vi "Pressure_4_R2.vi"() -> ()   [LabVIEW 2020]
uses:
  Support/Controls/Cmd_Mouse Popup.ctl
  Support/Controls/Clst_Initialize Input.ctl
  Support/Controls/Clst_Result inspec.ctl
  Support/Controls/Cmd_Var Data IO.ctl
  Variables/Global_Cal Info.vi
panel:
  in  "설정온도(℃)":string
  in  "측정시간(분)":string
  in  "STD Measured":string[][](table) caption="데이터로거 지시값 (bar)"
  out "Resolution":string[][](table) caption="Spec"
  in  "지시형태":string(combo)="Check"
  in  "Spec 변경":bool
  in  "Random":bool
  out "Spec":string[][](table)
  out "제목":string
  out "에러 출력":errorcluster
  out "Condition":string[][](table)
  in  "최소눈금":string(combo)
  out "단위":string
  in  "Measured":string[][](table) caption="교정대상기기 지시값"
  out "Load?":bool
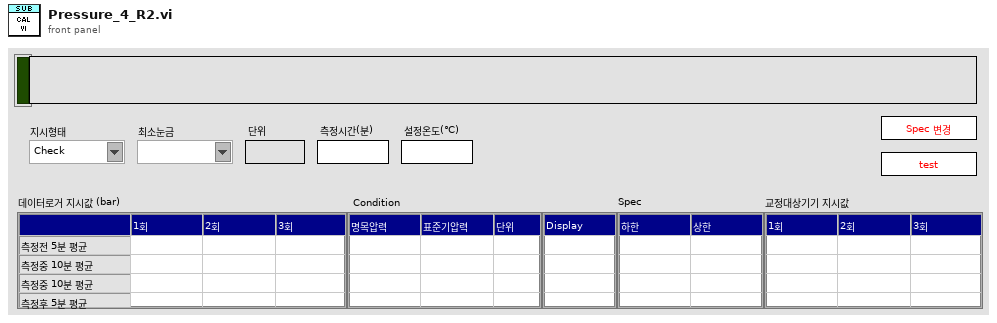
[diagram p1: front panel]
types:
  T1 = typedef "Cmd_Mouse Popup.ctl" = enum16{"활성화", "메뉴선택"}
  T2 = cluster{"Shift":bool, "Ctrl":bool, "Alt":bool, "Cmd":bool, "Opt":bool}
  T3 = typedef "Clst_Initialize Input.ctl" = cluster{"Initialize 1":cluster{"Condition":refnum<vi>[], "Spec":refnum<vi>[], "Measured":refnum<vi>[], "Resolution":refnum<vi>[], "Func_ext":string, "제목":refnum<vi>, "Measured_ADJ":refnum<vi>[]}, "Initialize 2":cluster{"문자열":refnum<vi>[], "콤보박스":refnum<vi>[], "링":refnum<vi>[], "열거형":refnum<vi>[], "테이블":refnum<vi>[], "여러열":refnum<vi>[], "디지털(DBL)":refnum<vi>[], "3D string":refnum<vi>[], "ctrl":refnum<vi>[], "boolean":refnum<vi>[]}}
  T4 = typedef "Clst_Result inspec.ctl" = cluster{"분해능":string, "문자열 1":string, "문자열 2":string, "숫자형 1":i32, "숫자형 2":i32, "숫자형 3":dbl, "문자배열 1D":string[], "문자배열 2D":string[][], "문자배열 3D":string[][][], "문자배열 4D":string[][][][], "불리언 1D":bool[]}
  T5 = typedef "Cmd_Var Data IO.ctl" = enum16{"Condition", "Condition Default", "Condition_Temp", "Resolution", "Resolution Default", "Resolution Old", "Spec", "Spec Default", "Spec Old", "Spec Temp", "Result", "Result2", "Result3", "Result_Temp", "Result_ADJ", "Result_ADJ2", "STD1", "STD2", "STD3", "STD4", "STD5", "STD Temp", "CMC", "CMC Default"}
  T6 = enum8{"Enabled", "Disabled", "Disabled and Grayed Out"}
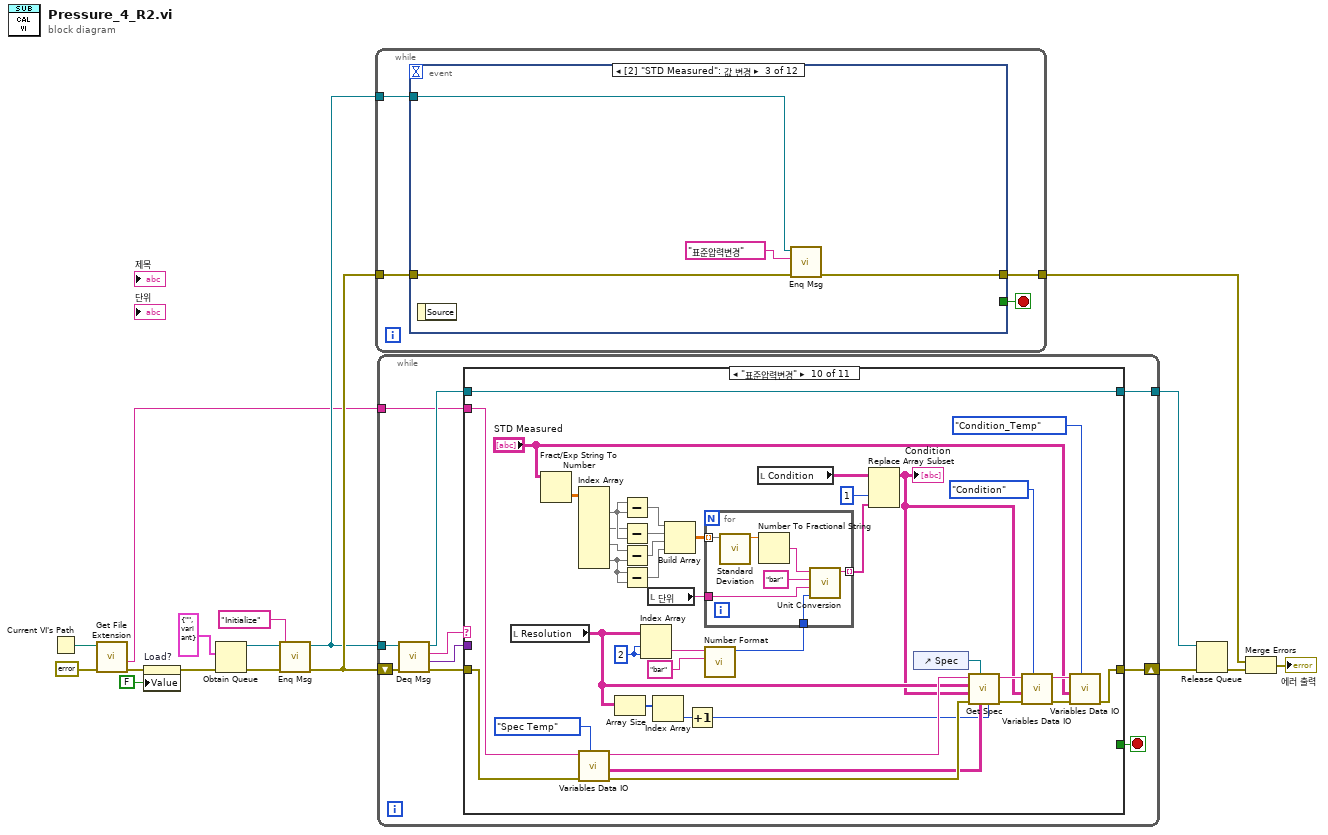
[diagram p0: block diagram]
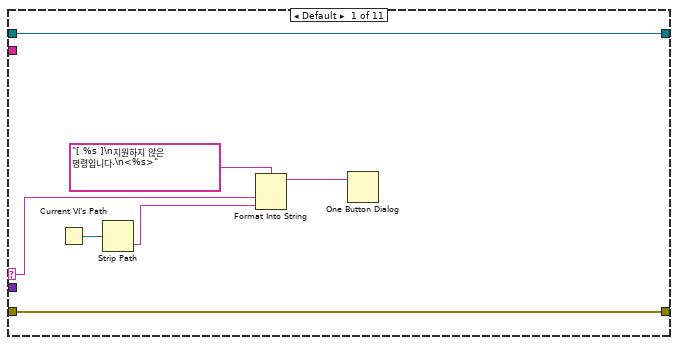
[diagram p2: hidden frame]
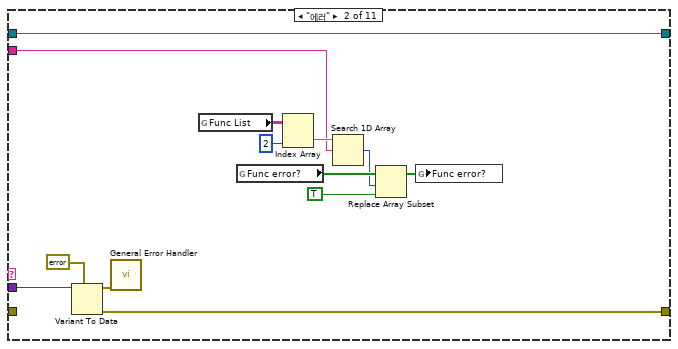
[diagram p3: hidden frame]
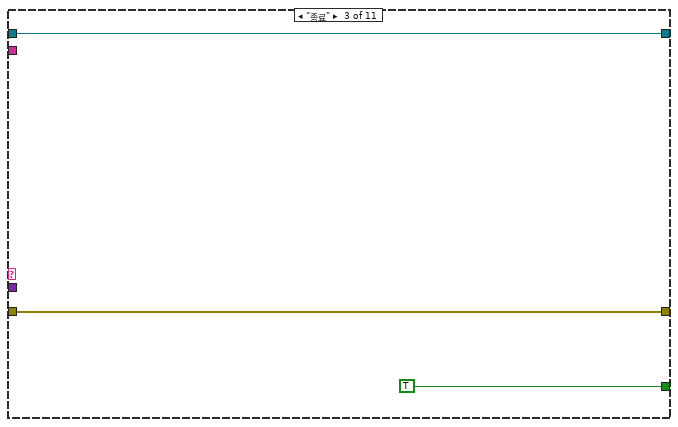
[diagram p4: hidden frame]
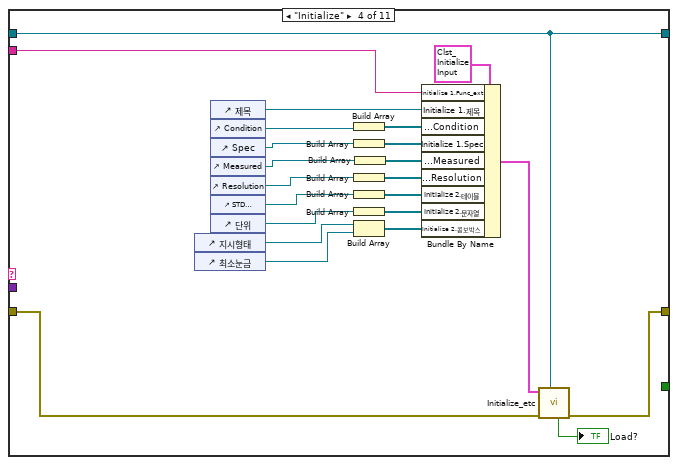
[diagram p5: hidden frame]
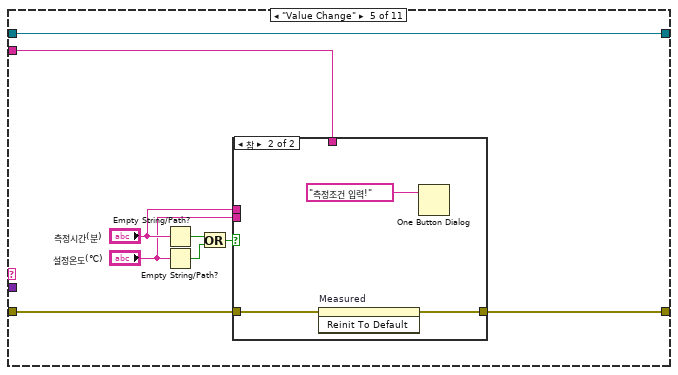
[diagram p6: hidden frame]
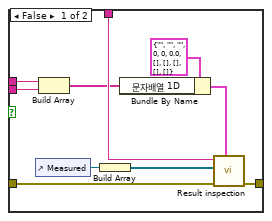
[diagram p7: hidden frame]
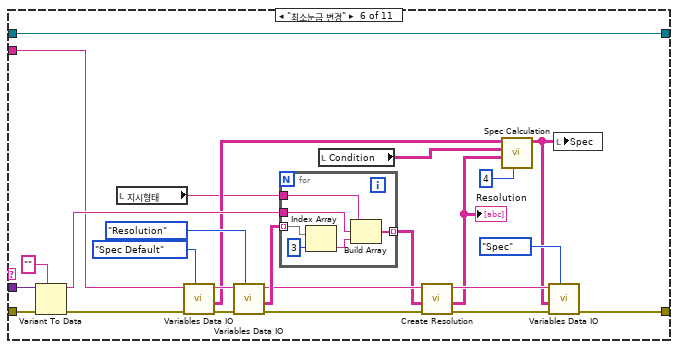
[diagram p8: hidden frame]
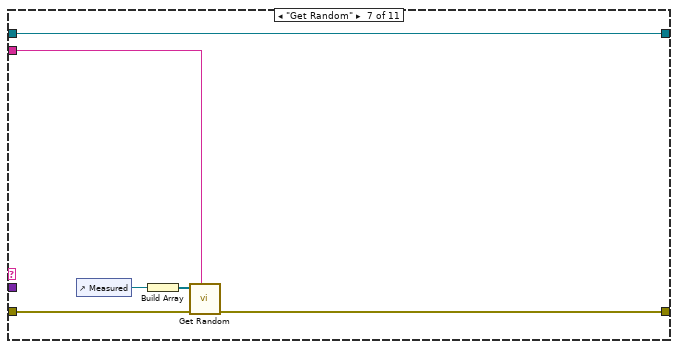
[diagram p9: hidden frame]
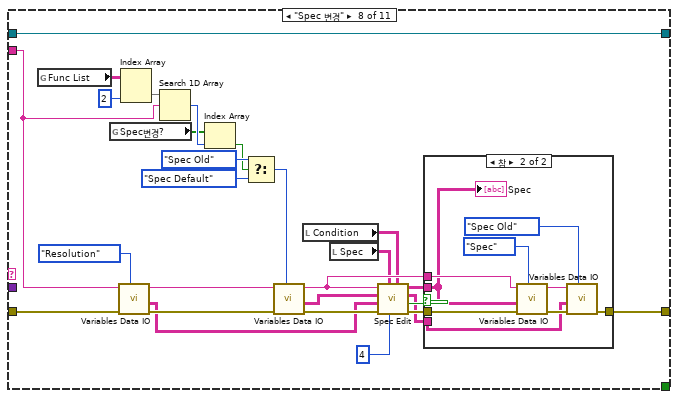
[diagram p10: hidden frame]
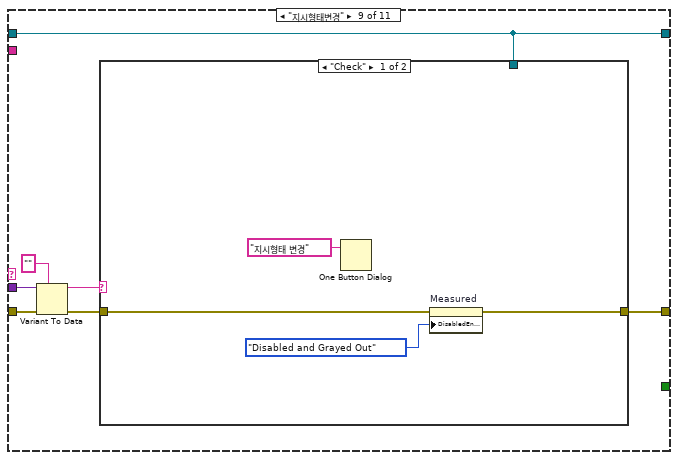
[diagram p12: hidden frame]
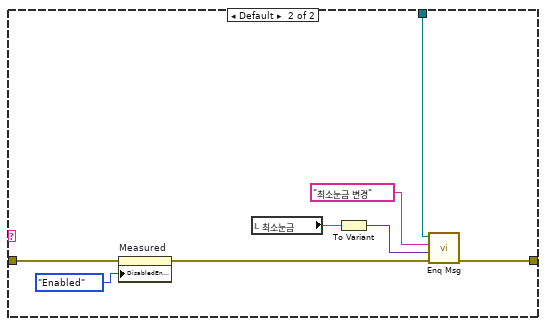
[diagram p13: hidden frame]
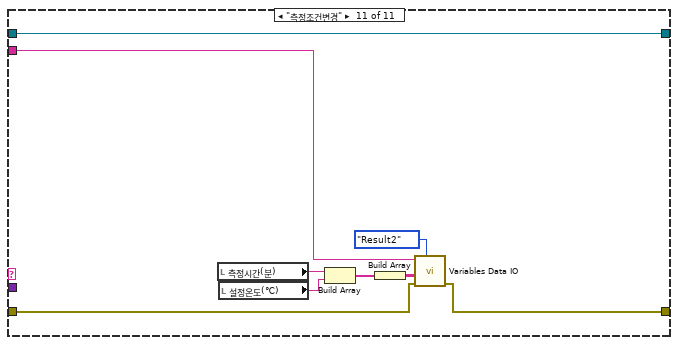
[diagram p14: hidden frame]
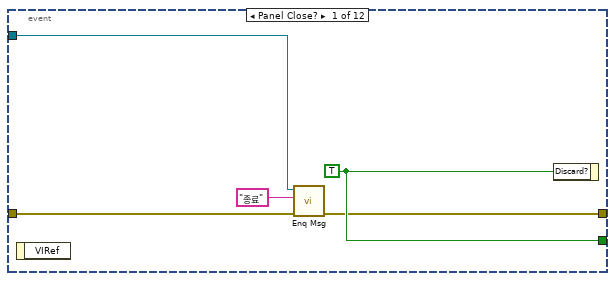
[diagram p15: hidden frame]
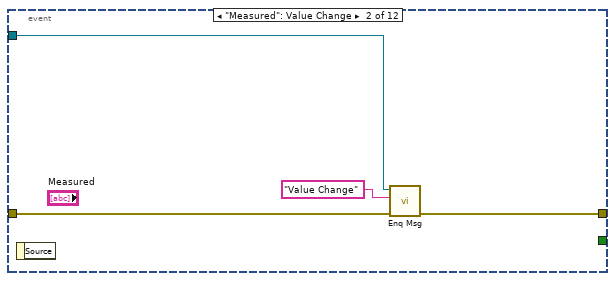
[diagram p16: hidden frame]
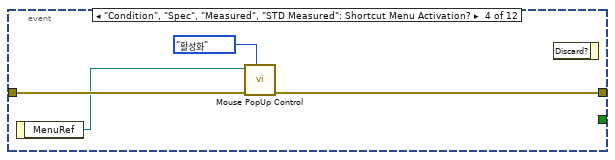
[diagram p17: hidden frame]
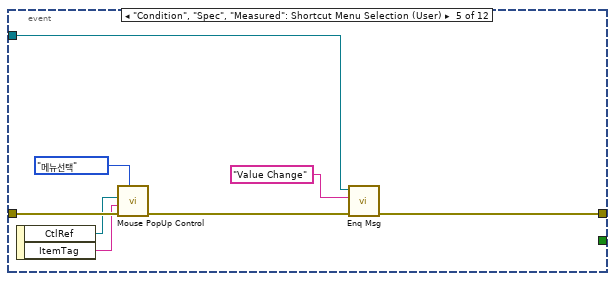
[diagram p18: hidden frame]
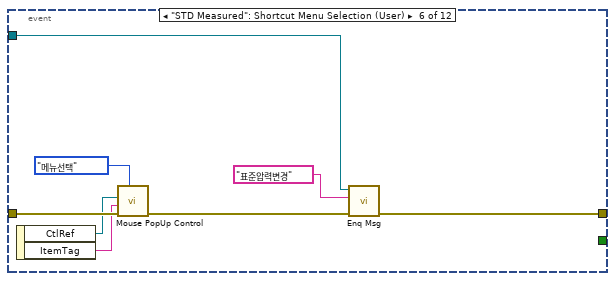
[diagram p19: hidden frame]
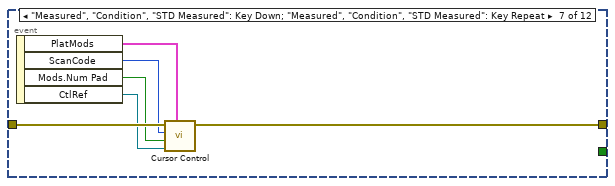
[diagram p20: hidden frame]
diagram:
  n1 = Current VI's Path() -> (path=w5:path)
  n2 = call <vilib>:"Get File Extension.vi"("error in (no error)"=errorcluster {"status"=FALSE, "code"=0, "source"=""} ("에러 상수"), "file"=w5) -> ("error out"=w3:errorcluster, "filename without extension"=w4:string)  [unwired: 5 in, 3 out]
  n3 = property on="Load?" class="Bool (엄격한)"(error in=w3, "Value"=FALSE ("Load?")) -> (error out=w2:errorcluster)  [unwired: 1 in, 1 out]
  n4 = Obtain Queue(element data type=cluster{"메세지":string, "값":variant} {"메세지"="", "값"=variant} ("Message Cluster"), error in (no error)=w2) -> (queue out=w14:refnum<queue>, error out=w16:errorcluster)  [unwired: 3 in, 1 out]
  n5 = call "Enq Msg.vi"("에러 입력(에러 없음)"=w16, "메세지"="Initialize", "큐 입력"=w14) -> ("에러 출력"=w15:errorcluster, "큐 출력"=w12:refnum<queue>)  [unwired: 7 in]
  n6 = while {
    tunnel: w15 -> [w19]
    tunnel: w12 -> [w20]
    tunnel: [w18] -> w9
    stop <- w21 stop-if-true
    n7 = event shown="[2] \"STD Measured\": 값 변경" {
      selector: _ -> [_ _ _ _ _ _ _ _ _ _ _ _]
      dyn-events: _ -> [_ _ _ _ _ _ _ _ _ _ _ _]
      timeout: _ -> [_ _ _ _ _ _ _ _ _ _ _ _]
      tunnel: [w26 _ _ _ _ _ _ _ _ _ _ _] -> w21
      tunnel: w20 -> [w24 w29 w33 _ w41 w49 _ w62 w68 w74 w82 w86]
      tunnel: w19 -> [w25 w30 w34 w37 w45 w53 w60 w63 w70 w76 w83 w85]
      tunnel: [w22 w28 w32 w36 w40 w48 w59 w61 w69 w75 w81 w84] -> w18
      event Panel Close? {
        w26 = TRUE ("버림?")
        n8 = event-data() -> ()  [unwired: 1 in, 1 out]
        n9 = call "Enq Msg.vi"("에러 입력(에러 없음)"=w25, "메세지"="종료", "큐 입력"=w24) -> ("에러 출력"=w22:errorcluster)  [unwired: 7 in, 1 out]
        n10 = event-data("Discard?"=w26) -> ()  [unwired: 1 in, 1 out]
      }
      event "Measured": Value Change {
        n11 = event-data() -> ()  [unwired: 1 in, 1 out]
        n12 = call "Enq Msg.vi"("에러 입력(에러 없음)"=w30, "메세지"="Value Change", "큐 입력"=w29) -> ("에러 출력"=w28:errorcluster)  [unwired: 7 in, 1 out]
      }
      event "STD Measured": Value Change {
        n13 = event-data() -> ()  [unwired: 1 in, 1 out]
        n14 = call "Enq Msg.vi"("에러 입력(에러 없음)"=w34, "메세지"="표준압력변경", "큐 입력"=w33) -> ("에러 출력"=w32:errorcluster)  [unwired: 7 in, 1 out]
      }
      event "Condition", "Spec", "Measured", "STD Measured": Shortcut Menu Activation? {
        n15 = event-data() -> ("MenuRef"=w35:refnum<k9>)  [unwired: 1 in]
        n16 = call "Mouse PopUp Control.vi"("type"=Cmd_Mouse_Popup."활성화", "error in"=w37, "메뉴 참조"=w35) -> ("error out"=w36:errorcluster)  [unwired: 8 in]
        n17 = event-data() -> ()  [unwired: 2 in, 1 out]
      }
      event "Condition", "Spec", "Measured": Shortcut Menu Selection (User) {
        n18 = event-data() -> ("CtlRef"=w43:refnum<vi>, "ItemTag"=w44:string)  [unwired: 1 in]
        n19 = call "Mouse PopUp Control.vi"("type"=Cmd_Mouse_Popup."메뉴선택", "error in"=w45, "아이템 태그"=w44, "Tbl 참조 번호"=w43) -> ("error out"=w42:errorcluster)  [unwired: 7 in]
        n20 = call "Enq Msg.vi"("에러 입력(에러 없음)"=w42, "메세지"="Value Change", "큐 입력"=w41) -> ("에러 출력"=w40:errorcluster)  [unwired: 7 in, 1 out]
      }
      event "STD Measured": Shortcut Menu Selection (User) {
        n21 = event-data() -> ("CtlRef"=w51:refnum<vi>, "ItemTag"=w52:string)  [unwired: 1 in]
        n22 = call "Mouse PopUp Control.vi"("type"=Cmd_Mouse_Popup."메뉴선택", "error in"=w53, "아이템 태그"=w52, "Tbl 참조 번호"=w51) -> ("error out"=w50:errorcluster)  [unwired: 7 in]
        n23 = call "Enq Msg.vi"("에러 입력(에러 없음)"=w50, "메세지"="표준압력변경", "큐 입력"=w49) -> ("에러 출력"=w48:errorcluster)  [unwired: 7 in, 1 out]
      }
      event "Measured", "Condition", "STD Measured": Key Down; "Measured", "Condition", "STD Measured": Key Repeat {
        n24 = event-data() -> ("PlatMods"=w55:T2, "ScanCode"=w58:i16, "Mods.Num Pad"=w57:bool, "CtlRef"=w56:refnum<vi>)  [unwired: 1 in]
        n25 = call "Cursor Control.vi"("플랫폼 조합키"=w55, "참조"=w56, "Num Pad"=w57, "ScanCode"=w58, "error in"=w60) -> ("error out"=w59:errorcluster)  [unwired: 5 in, 1 out]
      }
      event "Random": Value Change {
        n26 = event-data() -> ()  [unwired: 1 in, 1 out]
        n27 = call "Enq Msg.vi"("에러 입력(에러 없음)"=w63, "메세지"="Get Random", "큐 입력"=w62) -> ("에러 출력"=w65:errorcluster, "큐 출력"=w66:refnum<queue>)  [unwired: 7 in]
        n28 = call "Enq Msg.vi"("에러 입력(에러 없음)"=w65, "메세지"="Value Change", "큐 입력"=w66) -> ("에러 출력"=w61:errorcluster)  [unwired: 7 in, 1 out]
      }
      event "Spec 변경": Value Change {
        n29 = event-data() -> ()  [unwired: 1 in, 1 out]
        n30 = call "Enq Msg.vi"("에러 입력(에러 없음)"=w70, "메세지"="Spec 변경", "큐 입력"=w68) -> ("에러 출력"=w69:errorcluster)  [unwired: 7 in, 1 out]
      }
      event "지시형태": Value Change {
        n31 = event-data() -> ()  [unwired: 1 in, 1 out]
        n32 = To Variant(anything="지시형태") -> (Variant=w72:variant)
        n33 = call "Enq Msg.vi"("에러 입력(에러 없음)"=w76, "값"=w72, "메세지"="지시형태변경", "큐 입력"=w74) -> ("에러 출력"=w75:errorcluster)  [unwired: 6 in, 1 out]
      }
      event "최소눈금": Value Change {
        n34 = event-data() -> ()  [unwired: 1 in, 1 out]
        n35 = To Variant(anything="최소눈금") -> (Variant=w78:variant)
        n36 = call "Enq Msg.vi"("에러 입력(에러 없음)"=w83, "값"=w78, "메세지"="최소눈금 변경", "큐 입력"=w82) -> ("에러 출력"=w81:errorcluster)  [unwired: 6 in, 1 out]
      }
      event "측정시간(분)", "설정온도(℃)": Value Change {
        n37 = event-data() -> ()  [unwired: 1 in, 1 out]
        n38 = call "Enq Msg.vi"("에러 입력(에러 없음)"=w85, "메세지"="측정조건변경", "큐 입력"=w86) -> ("에러 출력"=w84:errorcluster)  [unwired: 7 in, 1 out]
      }
    }
  }
  n39 = while {
    shift-right: [w97] -> w11
    shift-left: w15 -> [w96]
    tunnel: w12 -> [w94]
    tunnel: [w89] -> w10
    tunnel: w4 -> [w88]
    stop <- w90 stop-if-true
    n40 = call "Deq Msg.vi"("에러 입력(에러 없음)"=w96, "큐 입력"=w94) -> ("에러 출력"=w95:errorcluster, "값"=w91:variant, "메세지"=w93:string, "큐 출력"=w92:refnum<queue>)  [unwired: 6 in]
    n41 = case shown="\"표준압력변경\"" w93 {
      selector: w93 -> [w100 _ _ _ _ _ _ _ _ _ _]
      tunnel: w95 -> [w104 _ w120 w128 w149 w188 w200 w223 w245 w276 w306]
      tunnel: [w104 w114 w120 w123 w151 w170 w197 w227 w246 w262 w305] -> w97
      tunnel: w92 -> [w103 w113 w118 w129 w152 w190 w202 w229 w240 w297 w313]
      tunnel: w91 -> [_ w115 _ _ _ w187 _ _ w243 _ _]
      tunnel: [_ _ TRUE ("버림?") _ _ _ _ _ _ _ _] -> w90
      tunnel: [w103 w113 w118 w129 w152 w190 w202 w229 w240 w297 w313] -> w89
      tunnel: w88 -> [_ w105 _ w124 w150 w180 w198 w204 _ w274 w307]
      frame Default {
        n42 = Current VI's Path() -> (path=w99:path)
        n43 = Strip Path(path=w99) -> (name=w98:string)  [unwired: 1 out]
        n44 = Format Into String(format string="[ %s ]\n지원하지 않은 명령입니다.\n<%s>" ("메시지"), w100, w98) -> (resulting string=w101:string)  [unwired: 2 in, 1 out]
        n45 = One Button Dialog(message=w101) -> ()  [unwired: 1 in, 1 out]
      }
      frame "에러" {
        n46 = Variant To Data(type=errorcluster {"status"=FALSE, "code"=0, "source"=""} ("에러 출력"), Variant=w115) -> (data=w117:errorcluster, error out=w114:errorcluster)  [unwired: 1 in]
        n47 = call <vilib>:"General Error Handler.vi"("error in (no error)"=w117) -> ()  [unwired: 10 in, 5 out]
        n48 = global read "Global_Cal Info.vi" "Func List"() -> (w111:string[][])
        n49 = global read "Global_Cal Info.vi" "Func error?"() -> (w108:bool[])
        n50 = Index Array(array=w111, index (col)=2 ("비활성화된 인덱스 (열)")) -> (element=w110:string[])  [unwired: 1 in]
        n51 = Search 1D Array(1D array=w110, element=w105) -> (index of element=w107:i32)  [unwired: 1 in]
        n52 = Replace Array Subset(array=w108, new element=TRUE ("새 원소/부분배열"), index=w107) -> (w106:bool[])
        n53 = global write "Global_Cal Info.vi" "Func error?"(w106) -> ()
      }
      frame "종료" {
      }
      frame "Initialize" {
        n54 = control-ref of="지시형태"() -> (w125:refnum<vi>)
        n55 = control-ref of="최소눈금"() -> (w135:refnum<vi>)
        n56 = control-ref of="제목"() -> (w133:refnum<vi>)
        n57 = control-ref of="Condition"() -> (w141:refnum<vi>)
        n58 = control-ref of="Spec"() -> (w131:refnum<vi>)
        n59 = control-ref of="Measured"() -> (w138:refnum<vi>)
        n60 = control-ref of="Resolution"() -> (w127:refnum<vi>)
        n61 = control-ref of="STD Measured"() -> (w121:refnum<vi>)
        n62 = control-ref of="단위"() -> (w132:refnum<vi>)
        n63 = Build Array(w141) -> (w140:refnum<vi>[])
        n64 = Build Array(w131) -> (w130:refnum<vi>[])
        n65 = Build Array(w127) -> (w126:refnum<vi>[])
        n66 = Build Array(w121) -> (w137:refnum<vi>[])
        n67 = Build Array(w132) -> (w136:refnum<vi>[])
        n68 = Build Array(w125, w135) -> (w134:refnum<vi>[])
        n69 = Build Array(w138) -> (w139:refnum<vi>[])
        n70 = Bundle By Name(cluster=T3 {"Initialize 1"={"Condition"=[], "Spec"=[], "Measured"=[], "Resolution"=[], "Func_ext"="", "제목"=refnum, "Measured_ADJ"=[]}, "Initialize 2"={"문자열"=[], "콤보박스"=[], "링"=[], "열거형"=[], "테이블"=[], "여러열"=[], "디지털(DBL)"=[], "3D string"=[], "ctrl"=[], "boolean"=[]}} ("입력 클러스터"), "Initialize 1.Func_ext"=w124, "Initialize 1.제목"=w133, "Initialize 1.Condition"=w140, "Initialize 1.Spec"=w130, "Initialize 1.Measured"=w139, "Initialize 1.Resolution"=w126, "Initialize 2.테이블"=w137, "Initialize 2.문자열"=w136, "Initialize 2.콤보박스"=w134) -> (w142:T3)
        n71 = call "Initialize_etc.vi"("큐 입력"=w129, "error in"=w128, "입력 클러스터"=w142) -> ("error out"=w123:errorcluster, "Load?"=→"Load?":bool)  [unwired: 6 in, 1 out]
      }
      frame "Value Change" {
        n72 = Empty String/Path?(string/path="측정시간(분)") -> (empty?=w147:bool)
        n73 = Empty String/Path?(string/path="설정온도(℃)") -> (empty?=w148:bool)
        n74 = Or(x=w147, y=w148) -> (x .or. y?=w146:bool)
        n75 = case shown="참" w146 {
          tunnel: [w162 w163] -> w151
          tunnel: w150 -> [w161 _]
          tunnel: w149 -> [w155 w164]
          tunnel: "측정시간(분)" -> [w154 _]
          tunnel: "설정온도(℃)" -> [w153 _]
          frame False {
            n76 = control-ref of="Measured"() -> (w160:refnum<vi>)
            n77 = Build Array(w154, w153) -> (w157:string[])
            n78 = Build Array(w160) -> (w159:refnum<vi>[])
            n79 = Bundle By Name(cluster=T4 {"분해능"="", "문자열 1"="", "문자열 2"="", "숫자형 1"=0, "숫자형 2"=0, "숫자형 3"=0.0, "문자배열 1D"=[], "문자배열 2D"=[], "문자배열 3D"=[], "문자배열 4D"=[], "불리언 1D"=[]} ("입력 클러스터"), "문자배열 1D"=w157) -> (w156:T4)
            n80 = call "Result inspection.vi"("입력 클러스터"=w156, "error in"=w155, "Ref. Data (Inspection)"=w159, "Func ext"=w161) -> ("error out"=w162:errorcluster)  [unwired: 4 in, 3 out]
          }
          frame True {
            n81 = invoke on="Measured" class="Tbl (엄격한)" method="Reinit To Default"(error in=w164) -> (error out=w163:errorcluster)  [unwired: 2 in, 2 out]
            n82 = One Button Dialog(message="측정조건 입력!" ("메시지")) -> ()  [unwired: 1 in, 1 out]
          }
        }
      }
      frame "최소눈금 변경" {
        n83 = Variant To Data(error in=w188, type="", Variant=w187) -> (data=w185:string, error out=w181:errorcluster)
        n84 = local read "지시형태"() -> (w166:string)
        n85 = call "Variables Data IO.vi"("Select"=Cmd_Var_Data_IO."Spec Default", "error in"=w181, "Func_ext"=w180) -> ("error out"=w178:errorcluster, "Data Out"=w176:string[][], "Func_ext Out"=w179:string)  [unwired: 6 in]
        n86 = call "Variables Data IO.vi"("Select"=Cmd_Var_Data_IO."Resolution", "error in"=w178, "Func_ext"=w179) -> ("error out"=w183:errorcluster, "Data Out"=w189:string[][], "Func_ext Out"=w182:string)  [unwired: 6 in]
        n87 = for {
          tunnel: w189 -> [w196] mode=indexing
          tunnel: w185 -> [w195]
          tunnel: [w193] -> w168 mode=indexing
          tunnel: w166 -> [w192]
          n88 = Index Array(array=w196, index=3 ("인덱스")) -> (element=w194:string)
          n89 = Build Array(w192, w195, w194) -> (w193:string[])
        }
        n90 = local read "Condition"() -> (w175:string[][])
        n91 = call "Create Resolution.vi"("에러 입력(에러 없음)"=w183, "Resolution"=w168, "Func_ext"=w182) -> ("에러 출력"=w171:errorcluster, "Resolution Out"=w167:string[][], "Func_ext 출력"=w172:string)  [unwired: 6 in]
        "Resolution" <- w167
        n92 = call "Spec Calculation.vi"("기준값 열번호"=4 ("열번호(기준값)"), "Resolution"=w167, "Condition in"=w175, "Spec Default"=w176) -> ("Spec out"=w169:string[][])  [unwired: 6 in, 1 out]
        n93 = call "Variables Data IO.vi"("Select"=Cmd_Var_Data_IO."Spec", "error in"=w171, "Data In"=w169, "Func_ext"=w172) -> ("error out"=w170:errorcluster)  [unwired: 5 in, 2 out]
        n94 = local write "Spec"(w169) -> ()
      }
      frame "Get Random" {
        n95 = control-ref of="Measured"() -> (w199:refnum<vi>)
        n96 = Build Array(w199) -> (w201:refnum<vi>[])
        n97 = call "Get Random.vi"("Func_Ext"=w198, "에러 입력"=w200, "Meas"=w201) -> ("에러 출력"=w197:errorcluster)  [unwired: 7 in, 1 out]
      }
      frame "Spec 변경" {
        n98 = global read "Global_Cal Info.vi" "Func List"() -> (w209:string[][])
        n99 = global read "Global_Cal Info.vi" "Spec변경?"() -> (w205:bool[])
        n100 = call "Variables Data IO.vi"("Select"=Cmd_Var_Data_IO."Resolution", "error in"=w223, "Func_ext"=w204) -> ("error out"=w222:errorcluster, "Data Out"=w216:string[][], "Func_ext Out"=w221:string)  [unwired: 6 in]
        n101 = Index Array(array=w209, index (col)=2 ("비활성화된 인덱스 (열)")) -> (element=w207:string[])  [unwired: 1 in]
        n102 = Search 1D Array(1D array=w207, element=w204) -> (index of element=w206:i32)  [unwired: 1 in]
        n103 = Index Array(array=w205, index=w206) -> (element=w210:bool)
        n104 = Select(t=Cmd_Var_Data_IO."Spec Old" ("Select"), s=w210, f=Cmd_Var_Data_IO."Spec Default" ("Select")) -> (s? t:f=w203:T5)
        n105 = call "Variables Data IO.vi"("Select"=w203, "error in"=w222, "Func_ext"=w221) -> ("error out"=w224:errorcluster, "Data Out"=w215:string[][], "Func_ext Out"=w217:string)  [unwired: 6 in]
        n106 = local read "Condition"() -> (w213:string[][])
        n107 = local read "Spec"() -> (w214:string[][])
        n108 = call "Spec Edit.vi"("Condition"=w213, "열번호(기준값)"=4 ("기준열(0)"), "Spec Value"=w214, "에러 입력(에러 없음)"=w224, "Resolution"=w216, "Spec Default"=w215, "Func_ext"=w217) -> ("에러 출력"=w228:errorcluster, "변경?"=w225:bool, "Spec Default out"=w219:string[][], "Spec 출력"=w226:string[][])  [unwired: 1 in]
        n109 = case shown="참" w225 {
          tunnel: w228 -> [w230 w238]
          tunnel: [w230 w234] -> w227
          tunnel: w226 -> [_ w236]
          tunnel: w217 -> [_ w237]
          tunnel: w219 -> [_ w232]
          frame False {
          }
          frame True {
            n110 = call "Variables Data IO.vi"("Select"=Cmd_Var_Data_IO."Spec", "error in"=w238, "Data In"=w236, "Func_ext"=w237) -> ("error out"=w235:errorcluster, "Func_ext Out"=w233:string)  [unwired: 5 in, 1 out]
            n111 = call "Variables Data IO.vi"("Select"=Cmd_Var_Data_IO."Spec Old", "error in"=w235, "Data In"=w232, "Func_ext"=w233) -> ("error out"=w234:errorcluster)  [unwired: 5 in, 2 out]
            "Spec" <- w236
          }
        }
      }
      frame "지시형태변경" {
        n112 = Variant To Data(error in=w245, type="", Variant=w243) -> (data=w241:string, error out=w244:errorcluster)
        n113 = case shown="\"Check\"" w241 {
          tunnel: w244 -> [w249 w257]
          tunnel: [w247 w253] -> w246
          tunnel: w240 -> [_ w251]
          frame "Check" {
            n114 = One Button Dialog(message="지시형태 변경" ("메시지")) -> ()  [unwired: 1 in, 1 out]
            n115 = property on="Measured" class="Tbl (엄격한)"(error in=w249, "DisabledEnum"=T6."Disabled and Grayed Out" ("비활성화")) -> (error out=w247:errorcluster)  [unwired: 1 in, 1 out]
          }
          frame Default {
            n116 = property on="Measured" class="Tbl (엄격한)"(error in=w257, "DisabledEnum"=T6."Enabled" ("비활성화")) -> (error out=w256:errorcluster)  [unwired: 1 in, 1 out]
            n117 = local read "최소눈금"() -> (w252:string)
            n118 = To Variant(anything=w252) -> (Variant=w255:variant)
            n119 = call "Enq Msg.vi"("에러 입력(에러 없음)"=w256, "값"=w255, "메세지"="최소눈금 변경", "큐 입력"=w251) -> ("에러 출력"=w253:errorcluster)  [unwired: 6 in, 1 out]
          }
        }
      }
      frame "표준압력변경" {
        w281 = 2 ("인덱스 (행)")
        n120 = local read "Resolution"() -> (w269:string[][])
        n121 = Fract/Exp String To Number(string="STD Measured") -> (number=w292:dbl[][])  [unwired: 3 in, 1 out]
        n122 = Index Array(array=w292) -> (element #1=w295:dbl[], element #2=w293:dbl[], element #3=w294:dbl[], element #4=w296:dbl[])  [unwired: 8 in]
        n123 = call "Variables Data IO.vi"("Select"=Cmd_Var_Data_IO."Spec Temp", "error in"=w276, "Func_ext"=w274) -> ("error out"=w275:errorcluster, "Data Out"=w272:string[][], "Func_ext Out"=w273:string)  [unwired: 6 in]
        n124 = Array Size(array=w269) -> (size(s)=w271:i32[])
        n125 = Subtract(x=w295, y=w295) -> (x-y=w291:dbl[])
        n126 = Subtract(x=w293, y=w295) -> (x-y=w290:dbl[])
        n127 = Subtract(x=w294, y=w296) -> (x-y=w289:dbl[])
        n128 = Subtract(x=w296, y=w296) -> (x-y=w288:dbl[])
        n129 = Index Array(array=w269, index (row)=w281, index (col)=w281) -> (element=w285:string)
        n130 = local read "단위"() -> (w286:string)
        n131 = Index Array(array=w271) -> (element=w270:i32)  [unwired: 1 in]
        n132 = Build Array(w291, w290, w289, w288) -> (w287:dbl[][])
        n133 = Increment(x=w270) -> (x+1=w268:i32)
        n134 = call "Number Format.vi"("입력단위"="bar", "입력값"=w285) -> ("정밀도(단위적용)"=w284:i32)  [unwired: 9 in]
        n135 = for {
          tunnel: w287 -> [w304] mode=indexing
          tunnel: w286 -> [w300]
          tunnel: [w299] -> w283 mode=indexing
          tunnel: w284 -> [w298]
          n136 = call "Standard Deviation.vi"("X"=w304) -> ("mean"=w303:dbl)  [unwired: 8 in, 2 out]
          n137 = Number To Fractional String(number=w303) -> (F-format string=w302:string)  [unwired: 3 in]
          n138 = call "Unit Conversion.vi"("소수점 자리수"=w298, "환산단위"=w300, "입력단위"="bar", "입력값"=w302) -> ("환산값 (string)"=w299:string)  [unwired: 2 in, 5 out]
        }
        n139 = local read "Condition"() -> (w278:string[][])
        n140 = Replace Array Subset(array=w278, new element=w283, index (col)=1 ("비활성화된 인덱스 (열)")) -> (w264:string[][])  [unwired: 1 in]
        "Condition" <- w264
        n141 = control-ref of="Spec"() -> (w279:refnum<vi>)
        n142 = call "Get Spec.vi"("NumRows"=w268, "Spec in"=w272, "Spec Ref."=w279, "error in"=w275, "Condition in"=w264, "Resolution in"=w269, "Func_ext"=w273) -> ("error out"=w267:errorcluster, "Func_ext Out"=w265:string)  [unwired: 3 out]
        n143 = call "Variables Data IO.vi"("Select"=Cmd_Var_Data_IO."Condition", "error in"=w267, "Data In"=w264, "Func_ext"=w265) -> ("error out"=w263:errorcluster, "Func_ext Out"=w260:string)  [unwired: 5 in, 1 out]
        n144 = call "Variables Data IO.vi"("Select"=Cmd_Var_Data_IO."Condition_Temp", "error in"=w263, "Data In"="STD Measured", "Func_ext"=w260) -> ("error out"=w262:errorcluster)  [unwired: 5 in, 2 out]
      }
      frame "측정조건변경" {
        n145 = local read "측정시간(분)"() -> (w311:string)
        n146 = local read "설정온도(℃)"() -> (w310:string)
        n147 = Build Array(w311, w310) -> (w309:string[])
        n148 = Build Array(w309) -> (w312:string[][])
        n149 = call "Variables Data IO.vi"("Select"=Cmd_Var_Data_IO."Result2", "error in"=w306, "Data In"=w312, "Func_ext"=w307) -> ("error out"=w305:errorcluster)  [unwired: 5 in, 2 out]
      }
    }
  }
  n150 = Release Queue(queue=w10, error in (no error)=w11) -> (error out=w8:errorcluster)  [unwired: 1 in, 2 out]
  n151 = Merge Errors(w9, w8) -> (→"에러 출력":errorcluster)
